vi "Graph.vi"(0 "Cluster":cluster{waveform(dbl)[], digitalwaveform[]}) -> ()   [LabVIEW 2015]
panel:
  out "Mixed Signal Graph 2":cluster{waveform(dbl)[], digitalwaveform[]}(graph)
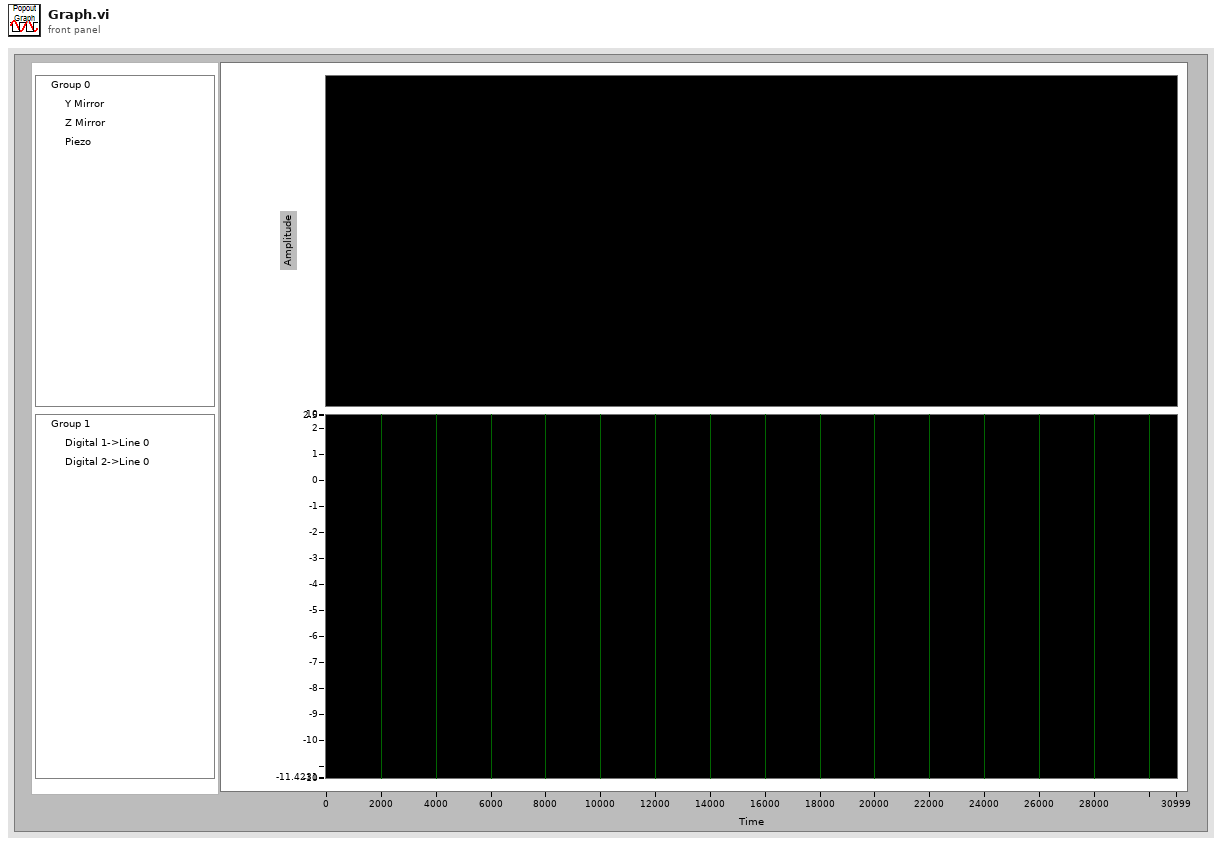
[diagram p1: front panel]
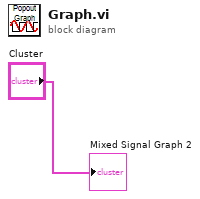
[diagram p0: block diagram]
diagram:
  "Mixed Signal Graph 2" <- "Cluster"
